vi "Read Di.vi"(0 "FPGA API in":refnum<class "FPGA API Mock.lvclass">, 11 "error in (no error)":errorcluster) -> (4 "FPGA API out":refnum<class "FPGA API Mock.lvclass">, 6 "DIs":bool[](array[boolean]), 15 "error out":errorcluster)   [LabVIEW 2019, in "FPGA API Mock.lvclass"]
uses:
  FPGA API Mock.lvclass
  FPGA API Mock.lvclass/FPGA API Mock.ctl
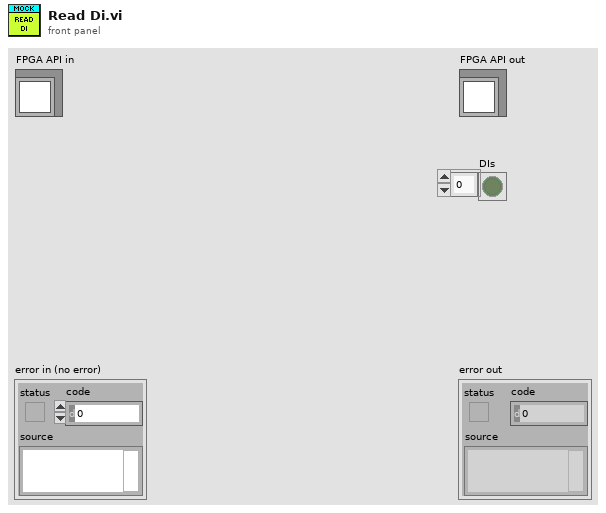
[diagram p1: front panel]
types:
  T1 = typedef "FPGA API Mock.lvclass/Data.ctl" = cluster{"DO":bool[], "DI":bool[], "AI":dbl[], "AO":dbl[]}
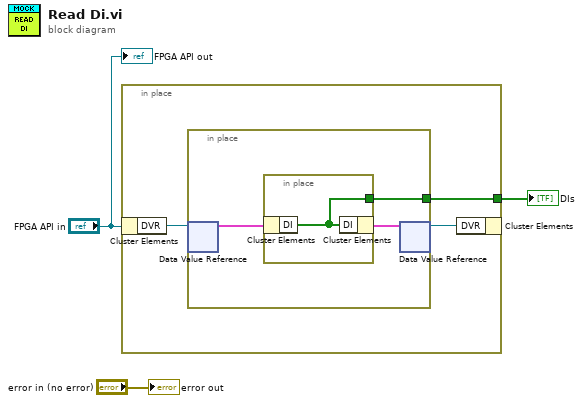
[diagram p0: block diagram]
diagram:
  n1 = in-place {
    in-place-border: [w4] -> w1
    n2 = in-place-cluster #1("FPGA API in") -> ("DVR"=w5:refnum<data-value>)
    n3 = in-place {
      in-place-border: [w7] -> w4
      n4 = in-place-dvr #2(w5) -> (w9:T1)  [unwired: 1 out]
      n5 = in-place {
        in-place-border: [w10] -> w7
        n6 = in-place-cluster #3(w9) -> ("DI"=w10:bool[])
        n7 = in-place-cluster #3("DI"=w10) -> (w8:T1)
      }
      n8 = in-place-dvr #2(w8) -> (w6:refnum<data-value>)  [unwired: 1 out]
    }
    n9 = in-place-cluster #1("DVR"=w6) -> ()  [unwired: 1 out]
  }
  "DIs" <- w1
  "error out" <- "error in (no error)"
  "FPGA API out" <- "FPGA API in"
